vi "Read Laser State.vi"(8 "error in (no error)":errorcluster, 11 "Laser Ethernet Rack in":refnum<class "Laser Ethernet Rack.lvclass">) -> (0 "error out":errorcluster, 2 "Cluster":T1, 3 "Laser Ethernet Rack out":refnum<class "Laser Ethernet Rack.lvclass">)   [LabVIEW 2023, in "Laser Ethernet Rack.lvclass"]
uses:
  Laser Ethernet Rack.lvclass
  Laser Ethernet Rack.lvclass/Laser Ethernet Rack.ctl
  laser_log_state.ctl
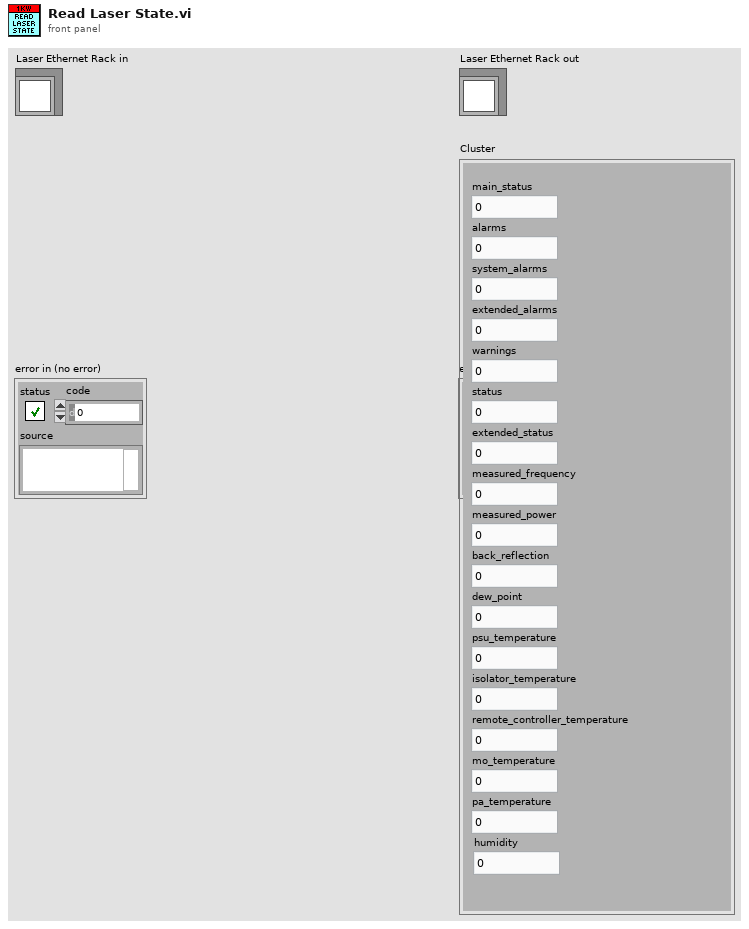
[diagram p1: front panel]
types:
  T1 = typedef "Laser Ethernet Rack.lvclass/laser_log_state.ctl" = cluster{"main_status":u32, "alarms":u32, "system_alarms":u32, "extended_alarms":u32, "warnings":u32, "status":u32, "extended_status":u32, "measured_frequency":sgl, "measured_power":sgl, "back_reflection":sgl, "dew_point":sgl, "psu_temperature":sgl, "isolator_temperature":sgl, "remote_controller_temperature":sgl, "mo_temperature":sgl, "pa_temperature":sgl, "humidity":sgl}
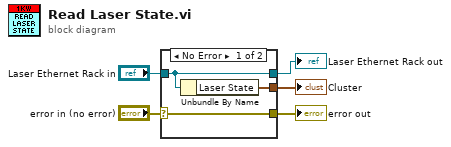
[diagram p0: block diagram]
diagram:
  n1 = case shown="No Error" "error in (no error)" {
    selector: "error in (no error)" -> [w8 w9]
    tunnel: [w8 w9] -> w4
    tunnel: [w7 w10] -> w2
    tunnel: "Laser Ethernet Rack in" -> [w7 w10]
    tunnel: [w6 _] -> w1
    frame No Error {
      n2 = Unbundle By Name(w7) -> ("Laser State"=w6:T1)
    }
    frame Error {
    }
  }
  "error out" <- w4
  "Laser Ethernet Rack out" <- w2
  "Cluster" <- w1
